vi "Wait For Exit.vi"(7 "timeout [ms] (1)":i32=1, 8 "error in":errorcluster, 11 "pipe in":T1) -> (0 "error out":errorcluster, 2 "exit code":i32, 3 "pipe out":T1)   [LabVIEW 2013, in "LV Process library.lvlib"]
doc: "Calls lv_proc.dll to wait for process exit. Be carefull using this with timeout set to 0 because it will hangup until process exit. It does not terminates the process, it only waits until it finishes. If process did not exited till the timeout error is generated.\n---\nLV Process works only with lv_proc.dll library, which is part of vipm package or should be delivered together with packed library. Placement of this dll is selected in terminal of Create Process.vi."
uses:
  LV Process library.lvlib
  Pipe Handle.ctl
panel:
  in  "code mem":i32
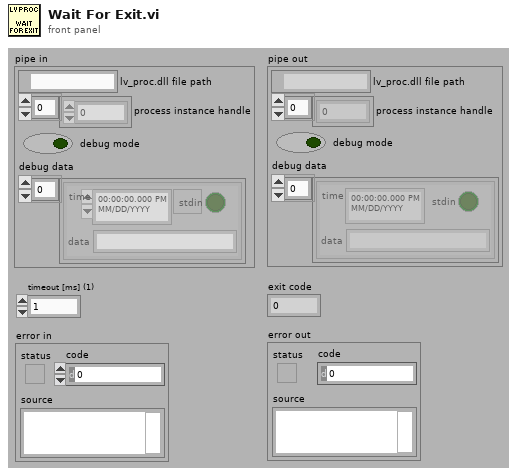
[diagram p1: front panel]
types:
  T1 = typedef "LV Process library.lvlib/Pipe Handle.ctl" = cluster{"lv_proc.dll file path":path, "process instance handle":u32[], "debug mode":bool, "debug data":cluster{"time":timestamp, "stdin":bool, "data":string}[]}
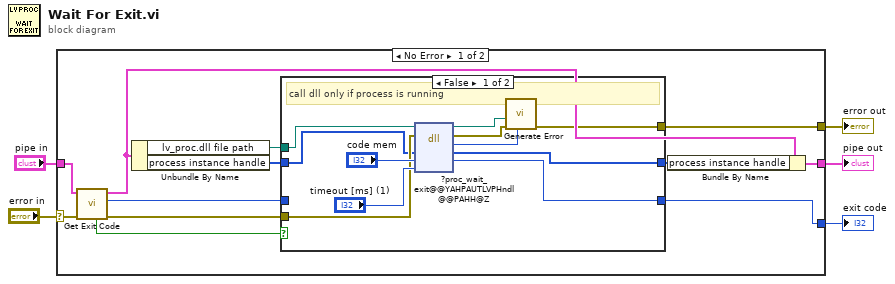
[diagram p0: block diagram]
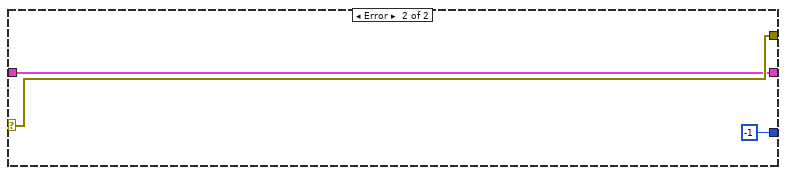
[diagram p3: hidden frame]
diagram:
  n1 = case shown="No Error" "error in" {
    selector: "error in" -> [w7 w34]
    tunnel: [w17 w34] -> w5
    tunnel: [w16 -1 ("code")] -> w4
    tunnel: [w14 w33] -> w3
    tunnel: "pipe in" -> [w12 w33]
    frame No Error {
      n2 = call "Get Exit Code.vi"("error in"=w7, "pipe in"=w12) -> ("error out"=w10:errorcluster, "exit code"=w8:i32, "pipe out"=w11:T1, "exited?"=w6:bool)  [unwired: 5 in, 1 out]
      n3 = Unbundle By Name(w11) -> ("lv_proc.dll file path"=w15:path, "process instance handle"=w9:u32[])
      n4 = case shown="False" w6 {
        tunnel: [w18 w31] -> w17
        tunnel: [w26 w29] -> w16
        tunnel: [w21 w30] -> w13
        tunnel: w10 -> [w25 w31]
        tunnel: w9 -> [w24 w30]
        tunnel: w8 -> [_ w29]
        tunnel: w15 -> [w23 _]
        frame False {
          # "call dll only if process is running"
          n5 = dll-call lib="C:/Data/GOLPI/LV Process/lv_proc.dll" fn="?proc_wait_exit@@YAHPAUTLVPHndl@@PAHH@Z" label="proc_wait_exit"(path in=w23, error in=w25, "proc"=w24, "code"="code mem", "timeout [ms]"="timeout [ms] (1)") -> (path out=w20:path, error out=w19:errorcluster, "error"=w22:i32, "proc"=w21:u32[], "code"=w26:i32)  [unwired: 2 in]
          n6 = call "Generate Error.vi"("error code in"=w22, "error in"=w19, "lv_proc.dll path in"=w20) -> ("error out"=w18:errorcluster)  [unwired: 6 in, 1 out]
        }
        frame True {
        }
      }
      n7 = Bundle By Name(cluster=w11, "process instance handle"=w13) -> (w14:T1)
    }
    frame Error {
    }
  }
  "error out" <- w5
  "exit code" <- w4
  "pipe out" <- w3
